vi "MB LRC-8.vi"(11 "String":string) -> (1 "LRC-8":u8, 2 "LRC-8":string, 3 "string & LRC-8":string)   [LabVIEW 2019, in "NI_modbus_upd.lvlib"]
uses:
  NI_modbus_upd.lvlib
panel:
  # "VI Name: MB LRC-8.vi\nPurpose: Computes the LRC of a string."
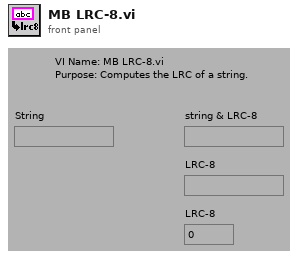
[diagram p1: front panel]
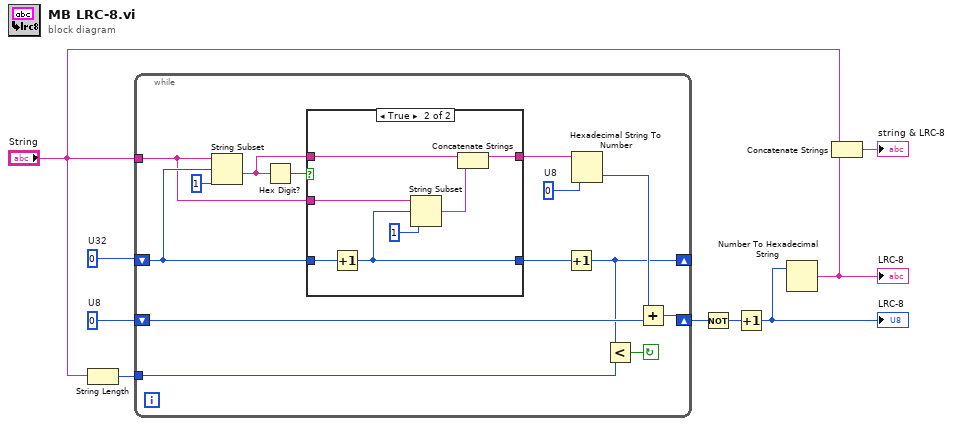
[diagram p0: block diagram]
diagram:
  w9 = u32 0  # U32
  w8 = u8 0  # U8
  n1 = String Length(string="String") -> (length=w7:i32)
  n2 = while {
    tunnel: "String" -> [w18]
    tunnel: w7 -> [w11]
    shift-left: w8 -> [w15]
    shift-right: [w14] -> w6
    shift-left: w9 -> [w22]
    shift-right: [w10] -> _
    stop <- w12 continue-if-true
    w17 = u8 0  # U8
    n3 = String Subset(string=w18, offset (0)=w22, length (rest)=1) -> (substring=w19:string)
    n4 = Hex Digit?(1:w19) -> (0:w20:bool)
    n5 = case shown="True" w20 {
      tunnel: w22 -> [w24 w32]
      tunnel: [w24 w30] -> w21
      tunnel: w19 -> [w25 w28]
      tunnel: w18 -> [_ w29]
      tunnel: [w25 w26] -> w16
      frame False {
      }
      frame True {
        n6 = Increment(x=w32) -> (x+1=w30:u32)
        n7 = String Subset(string=w29, offset (0)=w30, length (rest)=1) -> (substring=w27:string)
        n8 = Concatenate Strings(w28, w27) -> (w26:string)
      }
    }
    n9 = Increment(x=w21) -> (x+1=w10:u32)
    n10 = Hexadecimal String To Number(string=w16, default (0uL)=w17) -> (number=w13:u8)  [unwired: 1 in, 1 out]
    n11 = Less?(x=w10, y=w11) -> (x < y?=w12:bool)
    n12 = Add(x=w13, y=w15) -> (x+y=w14:u8)
  }
  n13 = Not(x=w6) -> (.not. x?=w5:u8)
  n14 = Increment(x=w5) -> (x+1=w4:u8)
  "LRC-8" <- w4
  n15 = Number To Hexadecimal String(2:w4) -> (0:w2:string)  [unwired: 1 in]
  "LRC-8" <- w2
  n16 = Concatenate Strings("String", w2) -> (→"string & LRC-8":string)
